vi "SVFA Phase Unit Conversion (1 Ch).vi"(0 "phase spectrum":cluster{"f0":dbl, "df":dbl, "phase":dbl[]} {"phase" format="%.2f"; "df" format="%.2f"; "f0" format="%.2f"}, 1 "desired units":T7(ring), 4 "spectrum info in":T1={"channel name"="", "description"="", "x-axis units"=0, "spectral info"={"spectrum type"=enum."Power [Magnitude^2]", "linear/dB"=enum."linear", "window"=0, "window size"=0, "FFT size"=0}, "engineering units"=1, "custom label"="", "dB reference [EU]"=0.0, "peak units"=enum."rms", "weighting filter"=0, "spectral density?"=FALSE, "unit label"="", "spectrum skewed?"=FALSE, "complimentary spectrum units"=enum."none"} {"x-axis units" items=["Time (s)"=0, "Frequency-CB (Hz)"=1, "Frequency-CPB (Hz)"=1248, "Frequency-Arbitrary (Hz)"=2357, "Quefrency (s)"=2, "Revolutions (rev)"=3, "Order"=4, "Speed (RPM)"=11, "Speed (rad/s)"=21, "Index"=65535]; "weighting filter" items=["Linear", "A-weighting", "B-weighting", "C-weighting", "ITU-R 468-4", "Dolby", "CCITT", "C-message", "Wb", "Wc", "Wd", "We", "Wf", "Wh", "Wj", "Wk", "Wm", "AES17 20 kHz lowpass", "AES17 40 kHz lowpass", "AES17 20 kHz highpass", "AES17 40 kHz highpass"]; "dB reference [EU]" format="%.2f"; "engineering units" items=["custom..."=0, "V"=1, "A"=21, "C"=30, "pC"=31, "s"=32, "-"=29, "Pa"=2, "N"=20, "g"=3, "m/s^2"=4, "m/s"=5, "m"=6, "mm/s"=12, "mm"=13, "micron/s"=14, "micron"=15, "in/s^2"=7, "in/s"=8, "in"=9, "mil/s"=10, "mil"=11, "rad/s^2"=16, "rad/s"=17, "rad"=18, "deg/s^2"=26, "deg/s"=27, "deg"=28, "RPM"=22, "cycle/s^2"=23, "Hz"=24, "cycle"=25, "strain"=19]; "spectral info"."window" items=["None "=0, "Hanning"=1, "Hamming"=2, "Blackman-Harris"=3, "Exact Blackman"=4, "Blackman"=5, "Flat Top"=6, "4 Term B-Harris "=7, "7 Term B-Harris"=8, "Low Sidelobe"=9, "Force - Exponential"=10, "Gaussian"=62]}, 5 "error in (no error)":errorcluster) -> (14 "converted phase spectrum":cluster{"f0":dbl, "df":dbl, "phase":dbl[]} {"phase" format="%.2f"; "df" format="%.2f"; "f0" format="%.2f"}, 15 "unit label":string, 18 "spectrum info out":T1={"channel name"="", "description"="", "x-axis units"=0, "spectral info"={"spectrum type"=enum."Power [Magnitude^2]", "linear/dB"=enum."linear", "window"=0, "window size"=0, "FFT size"=0}, "engineering units"=1, "custom label"="", "dB reference [EU]"=0.0, "peak units"=enum."rms", "weighting filter"=0, "spectral density?"=FALSE, "unit label"="", "spectrum skewed?"=FALSE, "complimentary spectrum units"=enum."none"} {"x-axis units" items=["Time (s)"=0, "Frequency-CB (Hz)"=1, "Frequency-CPB (Hz)"=1248, "Frequency-Arbitrary (Hz)"=2357, "Quefrency (s)"=2, "Revolutions (rev)"=3, "Order"=4, "Speed (RPM)"=11, "Speed (rad/s)"=21, "Index"=65535]; "weighting filter" items=["Linear", "A-weighting", "B-weighting", "C-weighting", "ITU-R 468-4", "Dolby", "CCITT", "C-message", "Wb", "Wc", "Wd", "We", "Wf", "Wh", "Wj", "Wk", "Wm", "AES17 20 kHz lowpass", "AES17 40 kHz lowpass", "AES17 20 kHz highpass", "AES17 40 kHz highpass"]; "dB reference [EU]" format="%.2f"; "engineering units" items=["custom..."=0, "V"=1, "A"=21, "C"=30, "pC"=31, "s"=32, "-"=29, "Pa"=2, "N"=20, "g"=3, "m/s^2"=4, "m/s"=5, "m"=6, "mm/s"=12, "mm"=13, "micron/s"=14, "micron"=15, "in/s^2"=7, "in/s"=8, "in"=9, "mil/s"=10, "mil"=11, "rad/s^2"=16, "rad/s"=17, "rad"=18, "deg/s^2"=26, "deg/s"=27, "deg"=28, "RPM"=22, "cycle/s^2"=23, "Hz"=24, "cycle"=25, "strain"=19]; "spectral info"."window" items=["None "=0, "Hanning"=1, "Hamming"=2, "Blackman-Harris"=3, "Exact Blackman"=4, "Blackman"=5, "Flat Top"=6, "4 Term B-Harris "=7, "7 Term B-Harris"=8, "Low Sidelobe"=9, "Force - Exponential"=10, "Gaussian"=62]}, 19 "error out":errorcluster)   [LabVIEW 2017]
doc: "Converts phase spectra between degrees, radians, and cycles. Wire data to the <B>phase spectrum</B> input to determine the polymorphic instance to use or manually select the instance."
uses:
  <vilib>/addons/_NISVFA/_Shared subVIs/Controls/svc_Spectrum Info.ctl
  <vilib>/addons/_NISVFA/_Shared subVIs/Controls/svc_X-Axis Units.ctl
  <vilib>/addons/_NISVFA/_Shared subVIs/Controls/svc_Spectrum Type.ctl
  <vilib>/addons/_NISVFA/_Shared subVIs/Controls/svc_Engineering Units Text Ring.ctl
  <vilib>/addons/_NISVFA/_Shared subVIs/Controls/svc_Weighting Filter Text Ring.ctl
  <vilib>/addons/_NISVFA/_Shared subVIs/Controls/svc_Complimentary Spectrum Units.ctl
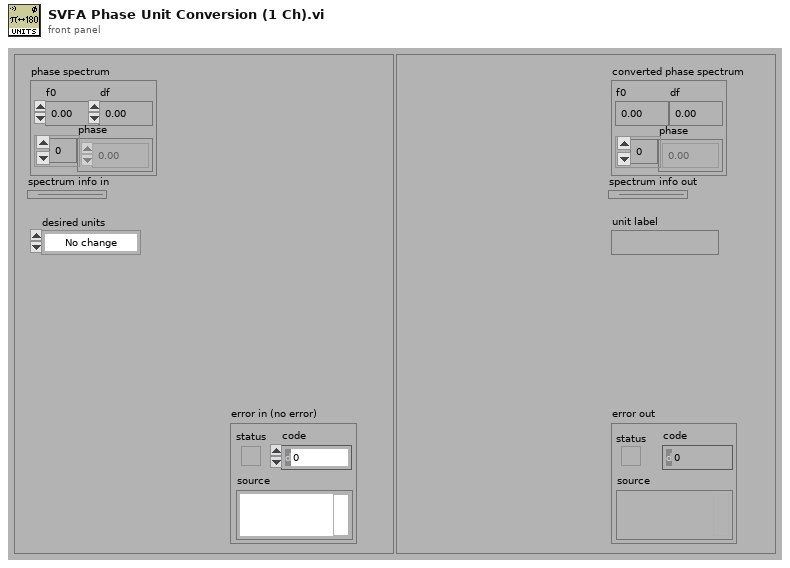
[diagram p1: front panel]
types:
  T1 = typedef "svc_Spectrum Info.ctl" = cluster{"channel name":string, "description":string, "x-axis units":T2, "spectral info":cluster{"spectrum type":T3, "linear/dB":enum16{"linear", "dB"}, "window":u16, "window size":i32, "FFT size":i32}, "engineering units":T4, "custom label":string, "dB reference [EU]":dbl, "peak units":enum16{"rms", "peak", "peak-peak"}, "weighting filter":T5, "spectral density?":bool, "unit label":string, "spectrum skewed?":bool, "complimentary spectrum units":T6}
  T2 = typedef "svc_X-Axis Units.ctl" = u16
  T3 = typedef "svc_Spectrum Type.ctl" = enum16{"FFT Spectrum [complex]", "Amplitude [Magnitude]", "Power [Magnitude^2]", "Cross Spectrum [complex]", "Frequency Response [Complex]"}
  T4 = typedef "svc_Engineering Units Text Ring.ctl" = u16
  T5 = typedef "svc_Weighting Filter Text Ring.ctl" = u16
  T6 = typedef "svc_Complimentary Spectrum Units.ctl" = enum16{"none", "radians", "degrees", "cycles", "imaginary"}
  T7 = enum16{"No change", "Radians", "Degrees", "Cycles"}
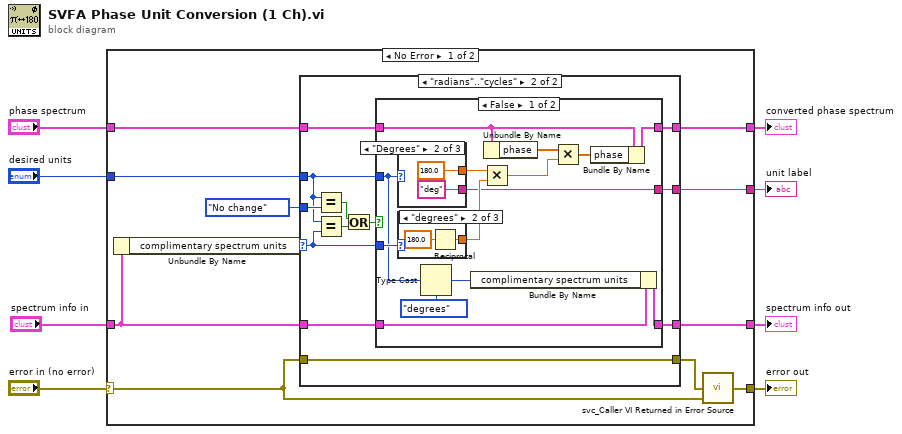
[diagram p0: block diagram]
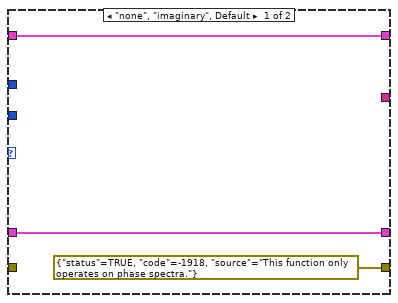
[diagram p2: hidden frame]
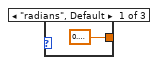
[diagram p3: hidden frame]
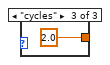
[diagram p4: hidden frame]
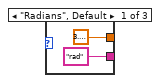
[diagram p5: hidden frame]
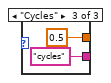
[diagram p6: hidden frame]
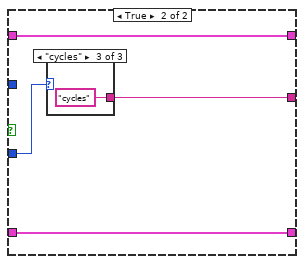
[diagram p7: hidden frame]
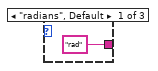
[diagram p8: hidden frame]
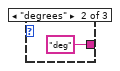
[diagram p9: hidden frame]
diagram:
  n1 = case shown="No Error" "error in (no error)" {
    selector: "error in (no error)" -> [w12 w67]
    tunnel: "phase spectrum" -> [w19 w68]
    tunnel: [w18 w68] -> w7
    tunnel: [w13 w67] -> w5
    tunnel: "desired units" -> [w17 _]
    tunnel: "spectrum info in" -> [w16 w66]
    tunnel: [w15 w66] -> w2
    tunnel: [w11 _] -> w1
    frame No Error {
      n2 = Unbundle By Name(w16) -> ("complimentary spectrum units"=w10:T6)
      n3 = case shown="\"radians\"..\"cycles\"" w10 {
        selector: w10 -> [_ w31]
        tunnel: w19 -> [w22 w33]
        tunnel: [w22 w32] -> w18
        tunnel: w17 -> [_ w24]
        tunnel: w16 -> [w21 w30]
        tunnel: [w21 w29] -> w15
        tunnel: [errorcluster {"status"=TRUE, "code"=-1918, "source"="This function only operates on phase spectra."} ("error in (no error)") w28] -> w14
        tunnel: w12 -> [_ w28]
        tunnel: [_ w27] -> w11
        tunnel: T7."No change" ("y") -> [_ w25]
        frame "none", "imaginary", Default {
        }
        frame "radians".."cycles" {
          n4 = Equal?(x=w24, y=w25) -> (x = y?=w23:bool)
          n5 = Equal?(x=w24, y=w31) -> (x = y?=w34:bool)
          n6 = Or(x=w23, y=w34) -> (x .or. y?=w26:bool)
          n7 = case shown="False" w26 {
            tunnel: w33 -> [w42 w62]
            tunnel: [w43 w62] -> w32
            tunnel: w24 -> [w37 _]
            tunnel: w31 -> [w46 w59]
            tunnel: w30 -> [w41 w61]
            tunnel: [w40 w61] -> w29
            tunnel: [w35 w60] -> w27
            frame False {
              n8 = case shown="\"Degrees\"" w37 {
                tunnel: [3.141592653589793 ("Pi") 180.0 0.5] -> w45
                tunnel: ["rad" ("unit label") "deg" ("unit label") "cycles" ("unit label")] -> w35
                frame "Radians", Default {
                }
                frame "Degrees" {
                }
                frame "Cycles" {
                }
              }
              n9 = case shown="\"degrees\"" w46 {
                tunnel: [0.3183098861837907 ("Reciprocal Of Pi") w50 2.0] -> w44
                frame "radians", Default {
                }
                frame "degrees" {
                  n10 = Reciprocal(x=180.0) -> (1/x=w50:dbl)
                }
                frame "cycles" {
                }
              }
              n11 = Type Cast(type=svc_Complimentary_Spectrum_Units."degrees" ("complimentary spectrum units"), x=w37) -> (*(type *) &x=w36:T6)
              n12 = Bundle By Name(cluster=w41, "complimentary spectrum units"=w36) -> (w40:T1)
              n13 = Multiply(x=w45, y=w44) -> (x*y=w39:dbl)
              n14 = Unbundle By Name(w42) -> ("phase"=w48:dbl[])
              n15 = Multiply(x=w48, y=w39) -> (x*y=w47:dbl[])
              n16 = Bundle By Name(cluster=w42, "phase"=w47) -> (w43:cluster{"f0":dbl, "df":dbl, "phase":dbl[]})
            }
            frame True {
              n17 = case shown="\"cycles\"" w59 {
                tunnel: ["rad" ("unit label") "deg" ("unit label") "cycles" ("unit label")] -> w60
                frame "radians", Default {
                }
                frame "degrees" {
                }
                frame "cycles" {
                }
              }
            }
          }
        }
      }
      n18 = call <vilib>:"svc_Caller VI Returned in Error Source.vi"("warning input to caller"=w12, "error in (no error)"=w14) -> ("error out"=w13:errorcluster)  [unwired: 3 in]
    }
    frame Error {
    }
  }
  "converted phase spectrum" <- w7
  "error out" <- w5
  "spectrum info out" <- w2
  "unit label" <- w1
